vi "FLOW-BUS RW.vi"(0 "VISA resource name":refnum<visa-resource-name>, 7 "FLOW-BUS Command Settings":T1={"Node Address (3)"=3, "Communication Command"=enum."Send parameter with destination address", "Process (0)"=0, "Parameter (0)"=0, "Data Type (0: Character)"=enum."Integer", "Data for Char, Int, or Long (0)"=0, "Data for Float (0)"=0.0, "Data for String"="", "Length of Requested String (0)"=0} {"Data Type (0: Character)" format="%0d"; "Communication Command" format="%0d"; "Node Address (3)" min=3 max=128}, 11 "error in (no error)":errorcluster {"code" format="%x"}) -> (4 "VISA resource name out":refnum<visa-resource-name>, 6 "Requested Char, Int or Long":u32, 8 "Requested Float or Long":sgl, 10 "Requested String":string, 15 "error out":errorcluster {"code" format="%x"})   [LabVIEW 2023, in "Bronkhorst FLOW-BUS.lvlib"]
doc: "This VI is the core of allmost all Bronkhorst FLOW-BUS Driver VI's. It is used to send FLOW-BUS commands to the selected instrument, and to decode the instruments response to those commands. Usages of this VI is as follows:\n\n - Wire up the VISA connections to their respective controls or constants.\n - To request a parameter (read), enter the values for the Node Address, Process, Parameter, and Data Type, and set the Communication Command to \"Request Parameter\"\n - To send a parameter (write), enter the values for the Node Address, Process, Parameter, Data Type, and the Data you want to send (in the Char/Int, Float/Long or String control) and set the Communication Command to \"Send paramter with destination address and 00 response\"\n- Now Run the VI"
uses:
  Bronkhorst FLOW-BUS.lvlib
  FLOW-BUS RW.ctl
panel:
  out "Formatted Command":string
  out "Received Response":string
  # "The process, parameter, and  data type values can be found in the parameter properties table on page 38 of document 9.17.027."
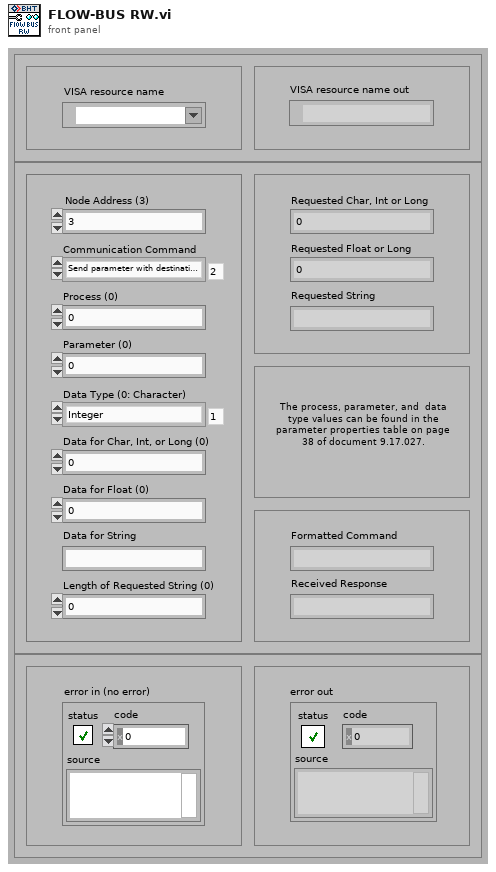
[diagram p1: front panel]
types:
  T1 = typedef "Bronkhorst FLOW-BUS.lvlib/FLOW-BUS RW.ctl" = cluster{"Node Address (3)":u8, "Communication Command":enum16{"Status message", "Send parameter with destination address and 00 response", "Send parameter with destination address", "Request parameter"}, "Process (0)":u16, "Parameter (0)":u16, "Data Type (0: Character)":enum16{"Character", "Integer", "Float or Long", "String"}, "Data for Char, Int, or Long (0)":u32, "Data for Float (0)":sgl, "Data for String":string, "Length of Requested String (0)":u8}
  T2 = enum16{"Status message", "Send parameter with destination address and 00 response", "Send parameter with destination address", "Request parameter"}
  T3 = enum16{"Character", "Integer", "Float or Long", "String"}
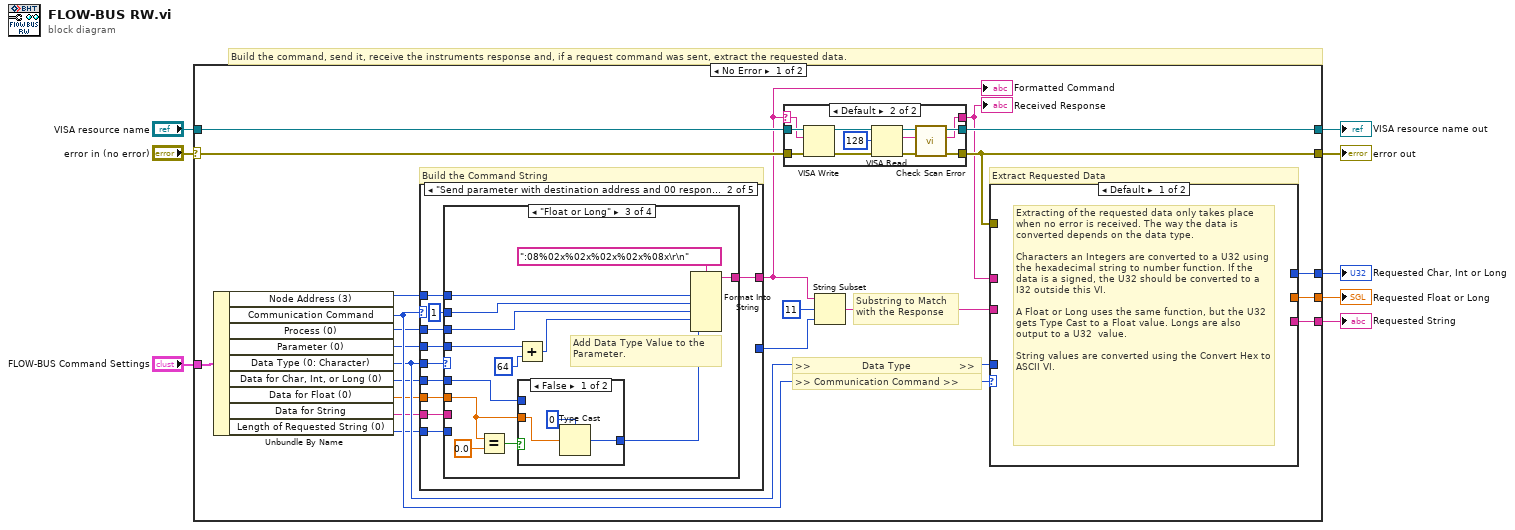
[diagram p0: block diagram]
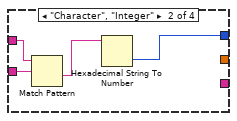
[diagram p5: hidden frame]
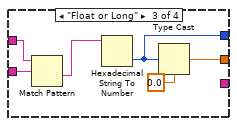
[diagram p6: hidden frame]
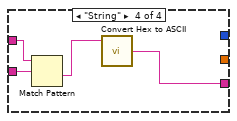
[diagram p7: hidden frame]
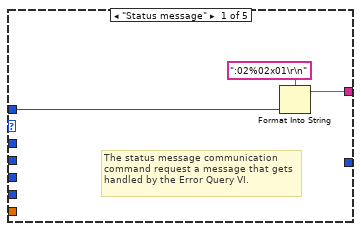
[diagram p8: hidden frame]
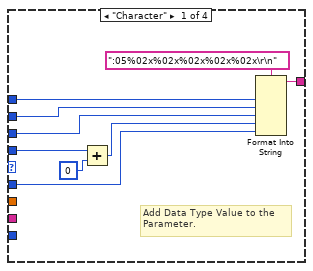
[diagram p9: hidden frame]
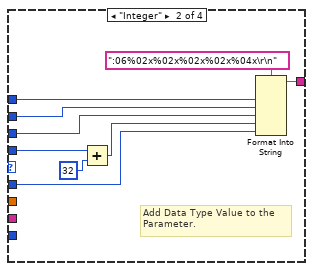
[diagram p10: hidden frame]
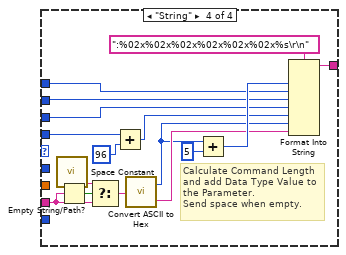
[diagram p12: hidden frame]
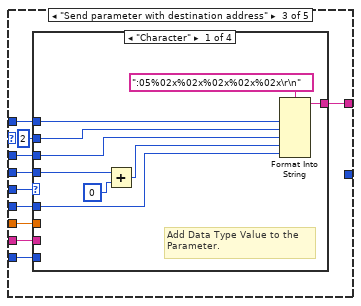
[diagram p13: hidden frame]
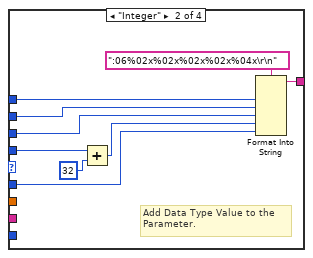
[diagram p14: hidden frame]
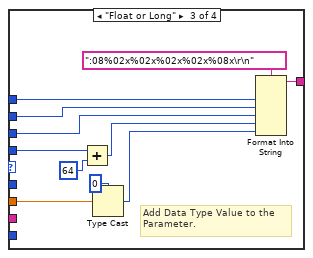
[diagram p15: hidden frame]
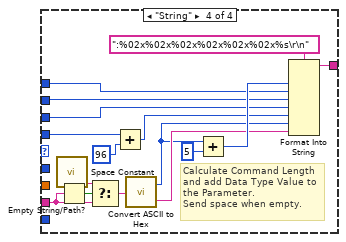
[diagram p16: hidden frame]
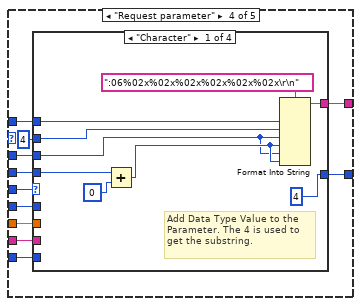
[diagram p17: hidden frame]
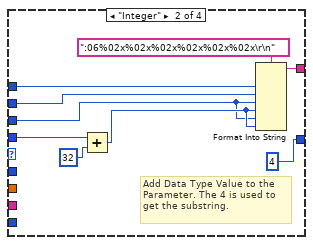
[diagram p18: hidden frame]
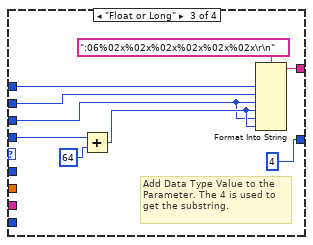
[diagram p19: hidden frame]
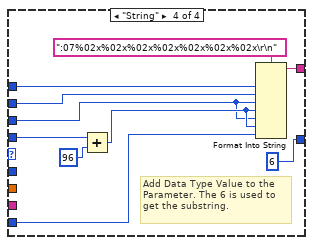
[diagram p20: hidden frame]
diagram:
  # "Build the command, send it, receive the instruments response and, if a request command was sent, extract the requested data."
  n1 = case shown="No Error" "error in (no error)" {
    selector: "error in (no error)" -> [w24 w241]
    tunnel: [w13 _] -> w8
    tunnel: [w12 w241] -> w7
    tunnel: [w15 _] -> w6
    tunnel: [w14 _] -> w5
    tunnel: [w28 w242] -> w4
    tunnel: "VISA resource name" -> [w23 w242]
    tunnel: "FLOW-BUS Command Settings" -> [w22 _]
    frame No Error {
      # "Extract Requested Data"
      # "Substring to Match\nwith the Response"
      # ">> Communication Command >>"
      # ">>                 Data Type                >>"
      # "Build the Command String"
      n2 = Unbundle By Name(w22) -> ("Node Address (3)"=w27:u8, "Communication Command"=w30:T2, "Process (0)"=w26:u16, "Parameter (0)"=w25:u16, "Data Type (0: Character)"=w29:T3, "Data for Char, Int, or Long (0)"=w21:u32, "Data for Float (0)"=w20:sgl, "Data for String"=w19:string, "Length of Requested String (0)"=w18:u8)
      n3 = case shown="\"Send parameter with destination address and 00 response\"" w30 {
        tunnel: w27 -> [w74 w80 w141 w197 _]
        tunnel: w26 -> [_ w81 w142 w198 _]
        tunnel: w25 -> [_ w82 w143 w199 _]
        tunnel: w29 -> [_ w85 w146 w202 _]
        tunnel: w21 -> [_ w83 w144 w200 _]
        tunnel: w20 -> [_ w84 w145 w201 _]
        tunnel: [w73 w79 w140 w196 ""] -> w9
        tunnel: w19 -> [_ w77 w138 w195 _]
        tunnel: w18 -> [_ w78 w139 w194 _]
        tunnel: [_ _ _ w193 _] -> w16
        frame "Status message" {
          # "The status message communication command request a message that gets handled by the Error Query VI."
          n4 = Format Into String(format string=":02%02x01\r\n", w74) -> (resulting string=w73:string)  [unwired: 2 in, 1 out]
        }
        frame "Send parameter with destination address and 00 response" {
          n5 = case shown="\"Float or Long\"" w85 {
            tunnel: w84 -> [_ _ w105 _]
            tunnel: w83 -> [w87 w95 w104 _]
            tunnel: w82 -> [w90 w98 w111 w133]
            tunnel: w81 -> [w91 w99 w112 w129]
            tunnel: u8 1 -> [w86 w100 w113 w130]
            tunnel: w80 -> [w92 w101 w114 w131]
            tunnel: [w89 w97 w110 w132] -> w79
            tunnel: w78 -> [_ _ _ _]
            tunnel: w77 -> [_ _ _ w123]
            frame "Character" {
              # "Add Data Type Value to the Parameter."
              n6 = Add(x=w90, y=u16 0 ("Parameter")) -> (x+y=w93:u16)
              n7 = Format Into String(format string=":05%02x%02x%02x%02x%02x\r\n", w92, w86, w91, w93, w87) -> (resulting string=w89:string)  [unwired: 2 in, 1 out]
            }
            frame "Integer" {
              # "Add Data Type Value to the Parameter."
              n8 = Add(x=w98, y=u16 32 ("Parameter")) -> (x+y=w102:u16)
              n9 = Format Into String(format string=":06%02x%02x%02x%02x%04x\r\n", w101, w100, w99, w102, w95) -> (resulting string=w97:string)  [unwired: 2 in, 1 out]
            }
            frame "Float or Long" {
              # "Add Data Type Value to the Parameter."
              n10 = Equal?(x=w105, y=sgl 0.0) -> (x = y?=w108:bool)
              n11 = Add(x=w111, y=u16 64 ("Parameter")) -> (x+y=w115:u16)
              n12 = case shown="False" w108 {
                tunnel: [w119 w120] -> w106
                tunnel: w105 -> [w117 _]
                tunnel: w104 -> [_ w120]
                frame False {
                  n13 = Type Cast(type=u32 0, x=w117) -> (*(type *) &x=w119:u32)
                }
                frame True {
                }
              }
              n14 = Format Into String(format string=":08%02x%02x%02x%02x%08x\r\n", w114, w113, w112, w115, w106) -> (resulting string=w110:string)  [unwired: 2 in, 1 out]
            }
            frame "String" {
              # "Calculate Command Length and add Data Type Value to the Parameter.\nSend space when empty."
              n15 = call <vilib>:"Space Constant.vi"() -> ("String"=w121:string)
              n16 = Empty String/Path?(string/path=w123) -> (empty?=w124:bool)
              n17 = Select(t=w121, s=w124, f=w123) -> (s? t:f=w122:string)
              n18 = Add(x=w133, y=u16 96 ("Parameter")) -> (x+y=w128:u16)
              n19 = call "Convert ASCII to Hex.vi"("String In"=w122) -> ("Hex ASCII String Length"=w126:i32, "Hex ASCII String Out"=w127:string)
              n20 = Add(x=w126, y=5) -> (x+y=w135:i32)
              n21 = Format Into String(format string=":%02x%02x%02x%02x%02x%02x%s\r\n", w135, w131, w130, w129, w128, w126, w127) -> (resulting string=w132:string)  [unwired: 2 in, 1 out]
            }
          }
        }
        frame "Send parameter with destination address" {
          n22 = case shown="\"Character\"" w146 {
            tunnel: w145 -> [_ _ w166 _]
            tunnel: w144 -> [w148 w156 _ _]
            tunnel: w143 -> [w151 w159 w170 w188]
            tunnel: w142 -> [w152 w160 w171 w184]
            tunnel: u8 2 -> [w147 w161 w172 w185]
            tunnel: w141 -> [w153 w162 w173 w186]
            tunnel: [w150 w158 w169 w187] -> w140
            tunnel: w139 -> [_ _ _ _]
            tunnel: w138 -> [_ _ _ w177]
            frame "Character" {
              # "Add Data Type Value to the Parameter."
              n23 = Add(x=w151, y=u16 0 ("Parameter")) -> (x+y=w154:u16)
              n24 = Format Into String(format string=":05%02x%02x%02x%02x%02x\r\n", w153, w147, w152, w154, w148) -> (resulting string=w150:string)  [unwired: 2 in, 1 out]
            }
            frame "Integer" {
              # "Add Data Type Value to the Parameter."
              n25 = Add(x=w159, y=u16 32 ("Parameter")) -> (x+y=w163:u16)
              n26 = Format Into String(format string=":06%02x%02x%02x%02x%04x\r\n", w162, w161, w160, w163, w156) -> (resulting string=w158:string)  [unwired: 2 in, 1 out]
            }
            frame "Float or Long" {
              # "Add Data Type Value to the Parameter."
              n27 = Add(x=w170, y=u16 64 ("Parameter")) -> (x+y=w174:u16)
              n28 = Type Cast(type=0, x=w166) -> (*(type *) &x=w167:i32)
              n29 = Format Into String(format string=":08%02x%02x%02x%02x%08x\r\n", w173, w172, w171, w174, w167) -> (resulting string=w169:string)  [unwired: 2 in, 1 out]
            }
            frame "String" {
              # "Calculate Command Length and add Data Type Value to the Parameter.\nSend space when empty."
              n30 = call <vilib>:"Space Constant.vi"() -> ("String"=w178:string)
              n31 = Empty String/Path?(string/path=w177) -> (empty?=w179:bool)
              n32 = Select(t=w178, s=w179, f=w177) -> (s? t:f=w176:string)
              n33 = Add(x=w188, y=u16 96 ("Parameter")) -> (x+y=w183:u16)
              n34 = call "Convert ASCII to Hex.vi"("String In"=w176) -> ("Hex ASCII String Length"=w181:i32, "Hex ASCII String Out"=w182:string)
              n35 = Add(x=w181, y=5) -> (x+y=w190:i32)
              n36 = Format Into String(format string=":%02x%02x%02x%02x%02x%02x%s\r\n", w190, w186, w185, w184, w183, w181, w182) -> (resulting string=w187:string)  [unwired: 2 in, 1 out]
            }
          }
        }
        frame "Request parameter" {
          n37 = case shown="\"Character\"" w202 {
            tunnel: w201 -> [_ _ _ _]
            tunnel: w200 -> [_ _ _ _]
            tunnel: w199 -> [w210 w219 w228 w238]
            tunnel: w198 -> [w209 w218 w227 w237]
            tunnel: u8 4 -> [w208 w217 w226 w236]
            tunnel: w197 -> [w207 w216 w225 w235]
            tunnel: [w205 w214 w223 w233] -> w196
            tunnel: w195 -> [_ _ _ _]
            tunnel: w194 -> [_ _ _ w232]
            tunnel: [4 ("offset (0)") 4 ("offset (0)") 4 ("offset (0)") 6 ("offset (0)")] -> w193
            frame "Character" {
              # "Add Data Type Value to the Parameter. The 4 is used to get the substring."
              n38 = Add(x=w210, y=u16 0 ("Parameter")) -> (x+y=w211:u16)
              n39 = Format Into String(format string=":06%02x%02x%02x%02x%02x%02x\r\n", w207, w208, w209, w211, w209, w211) -> (resulting string=w205:string)  [unwired: 2 in, 1 out]
            }
            frame "Integer" {
              # "Add Data Type Value to the Parameter. The 4 is used to get the substring."
              n40 = Add(x=w219, y=u16 32 ("Parameter")) -> (x+y=w220:u16)
              n41 = Format Into String(format string=":06%02x%02x%02x%02x%02x%02x\r\n", w216, w217, w218, w220, w218, w220) -> (resulting string=w214:string)  [unwired: 2 in, 1 out]
            }
            frame "Float or Long" {
              # "Add Data Type Value to the Parameter. The 4 is used to get the substring."
              n42 = Add(x=w228, y=u16 64 ("Parameter")) -> (x+y=w229:u16)
              n43 = Format Into String(format string=":06%02x%02x%02x%02x%02x%02x\r\n", w225, w226, w227, w229, w227, w229) -> (resulting string=w223:string)  [unwired: 2 in, 1 out]
            }
            frame "String" {
              # "Add Data Type Value to the Parameter. The 6 is used to get the substring."
              n44 = Add(x=w238, y=u16 96 ("Parameter")) -> (x+y=w239:u16)
              n45 = Format Into String(format string=":07%02x%02x%02x%02x%02x%02x%02x\r\n", w235, w236, w237, w239, w237, w239, w232) -> (resulting string=w233:string)  [unwired: 2 in, 1 out]
            }
          }
        }
        frame Default {
          # "There are currently four command types that can be sent using this VI. The request parameter command, the send parameter with destination address (and 00 response) command, and the status message command.\n \nAll commands use the format into string function to format the entered data into the correct command. The format string depends on the data type, as shown in the different cases. \n\nThe Status message command only uses the node address."
        }
      }
      "Formatted Command" <- w9
      n46 = case shown="Default" w9 {
        selector: w9 -> [w31 w34]
        tunnel: [w33 w39] -> w28
        tunnel: w24 -> [w32 w38]
        tunnel: w23 -> [w33 w37]
        tunnel: [w32 w36] -> w12
        tunnel: [w31 w35] -> w10
        frame "" {
          # "Unsupported Command"
        }
        frame Default {
          n47 = VISA Write(VISA resource name=w37, write buffer=w34, error in (no error)=w38) -> (VISA resource name out=w40:refnum<visa-resource-name>, error out=w41:errorcluster)  [unwired: 1 out]
          n48 = VISA Read(VISA resource name=w40, byte count=u32 128, error in (no error)=w41) -> (VISA resource name out=w43:refnum<visa-resource-name>, read buffer=w44:string, error out=w45:errorcluster)  [unwired: 1 out]
          n49 = call "Check Scan Error.vi"("error in (no error)"=w45, "Response Input"=w44, "VISA resource name"=w43) -> ("error out"=w36:errorcluster, "Response Output"=w35:string, "VISA resource name out"=w39:refnum<visa-resource-name>)  [unwired: 6 in]
        }
      }
      "Received Response" <- w10
      n50 = String Subset(string=w9, offset (0)=11, length (rest)=w16) -> (substring=w11:string)
      n51 = case shown="Default" w30 {
        tunnel: [_ w48] -> w15
        tunnel: [_ w47] -> w14
        tunnel: [_ w46] -> w13
        tunnel: w12 -> [_ w49]
        tunnel: w10 -> [_ w52]
        tunnel: w11 -> [_ w51]
        tunnel: w29 -> [_ w50]
        frame Default {
          # "Extracting of the requested data only takes place when no error is received. The way the data is converted depends on the data type. \n\nCharacters an Integers are converted to a U32 using the hexadecimal string to number function. If the data is a signed, the U32 should be converted to a I32 outside this VI.\n\nA Float or Long uses the same function, but the U32 gets Type Cast to a Float value. Longs are also output to a U32  value.\n\nString values are converted using the Convert Hex to ASCII VI."
        }
        frame "Request parameter" {
          n52 = case shown="No Error" w49 {
            tunnel: [_ w58] -> w48
            tunnel: [_ w57] -> w47
            tunnel: [_ w56] -> w46
            tunnel: w52 -> [_ w55]
            tunnel: w50 -> [_ w54]
            tunnel: w51 -> [_ w53]
            frame Error {
            }
            frame No Error {
              n53 = case shown="Default" w54 {
                tunnel: w55 -> [_ w60 w65 w69]
                tunnel: [_ _ w67 _] -> w57
                tunnel: [_ _ _ w72] -> w58
                tunnel: [_ w62 w66 _] -> w56
                tunnel: w53 -> [_ w61 w64 w71]
                frame Default {
                  # "The substring is used to select where in the response the data is located. \n\nIf this is not used, and corrupt data is received and read from a fixed position, false values will be displayed in the indicators."
                }
                frame "Character", "Integer" {
                  n54 = Match Pattern(string=w60, regular expression=w61) -> (after substring=w59:string)  [unwired: 1 in, 3 out]
                  n55 = Hexadecimal String To Number(string=w59) -> (number=w62:u32)  [unwired: 2 in, 1 out]
                }
                frame "Float or Long" {
                  n56 = Match Pattern(string=w65, regular expression=w64) -> (after substring=w63:string)  [unwired: 1 in, 3 out]
                  n57 = Hexadecimal String To Number(string=w63) -> (number=w66:u32)  [unwired: 2 in, 1 out]
                  n58 = Type Cast(type=sgl 0.0, x=w66) -> (*(type *) &x=w67:sgl)
                }
                frame "String" {
                  n59 = Match Pattern(string=w69, regular expression=w71) -> (after substring=w70:string)  [unwired: 1 in, 3 out]
                  n60 = call "Convert Hex to ASCII.vi"("Hex String"=w70) -> ("ASCII String"=w72:string)  [unwired: 1 in]
                }
              }
            }
          }
        }
      }
    }
    frame Error {
    }
  }
  "VISA resource name out" <- w4
  "error out" <- w7
  "Requested Float or Long" <- w5
  "Requested String" <- w6
  "Requested Char, Int or Long" <- w8
